vi "Test Save GIF (Memory).vi"(8 "error in (no error)":errorcluster) -> (0 "error out":errorcluster, 3 "Pass?":bool)   [LabVIEW 2020]
uses:
  <vilib>/picture/picture.llb/imagedata.ctl
  G-Image/Image IO/Polymorphic VIs/Save JPG Image (Memory).vi/70fca071-aecc-49e6-b287-23b8a0d46a54.vi
  G-Image/Private/Result To Error.vi
  G-Image/Private/Get Image Data.vi
  G-Image/Private/ARGB To RGBA.vi
  G-Image/Private/Depth To Number Channels.vi
  G-Image/Image Processing/Indexed Color To True Color Image.vi
  <vilib>/Utility/error.llb/Error Cluster From Error Code.vi
  G-Image/G-Image.lvlib
  G-Image/Image IO/Controls/Dither Type.ctl
  0a31d6d2-376c-4628-95d1-524ecda838ee.vi
  G-Image/Image IO/Polymorphic VIs/Save GIF Image (Path).vi
  G-Image/Image IO/Polymorphic VIs/Load Image (Path).vi
panel:
  out "Array":cluster{string, "new picture":picture}[](array[cluster])
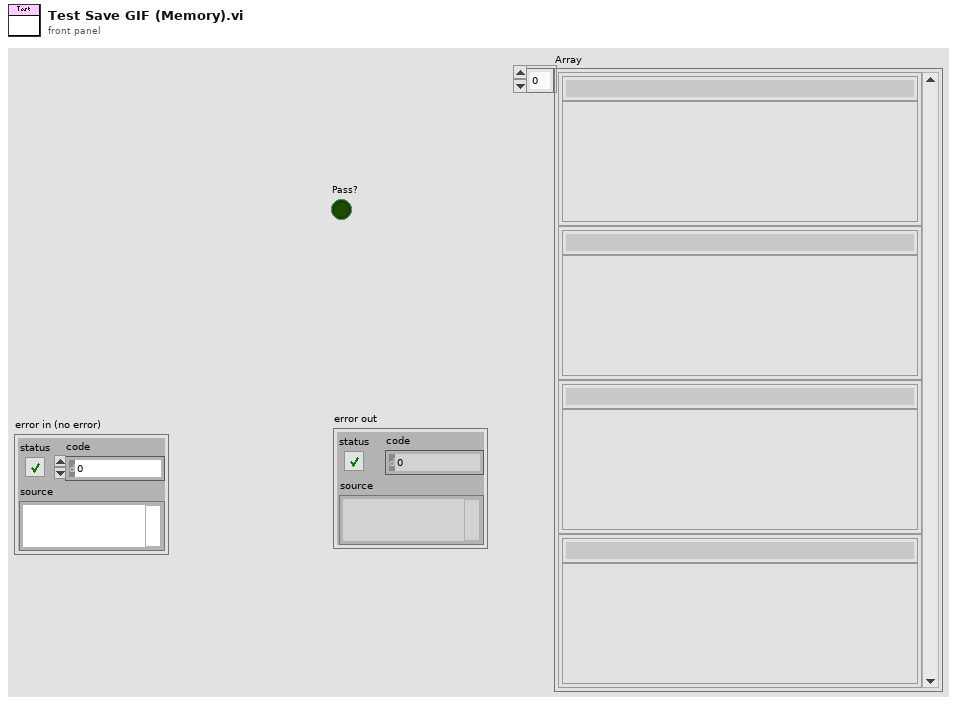
[diagram p1: front panel]
types:
  T1 = typedef "G-Image.lvlib/Dither Type.ctl" = enum32{"None", "Floyd-Steinberg"}
  T2 = typedef "imagedata.ctl" = cluster{"image type":i32, "image depth":i32, "image":u8[], "mask":u8[], "colors":u32[], "Rectangle":cluster{"left":i16, "top":i16, "right":i16, "bottom":i16}}
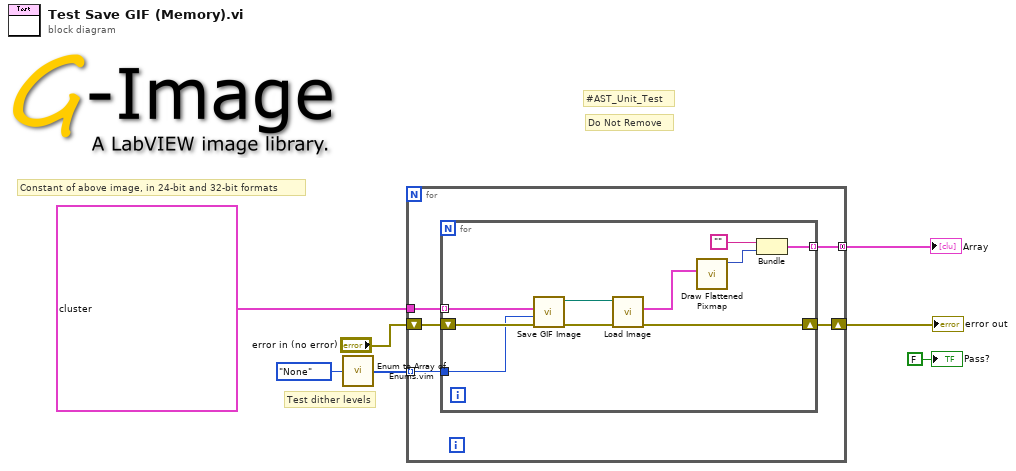
[diagram p0: block diagram]
diagram:
  # "Test dither levels"
  # "Constant of above image, in 24-bit and 32-bit formats"
  # "Do Not Remove"
  # "#AST_Unit_Test"
  n1 = call "Enum to Array of Enums.vim"("enum"=Dither_Type."None" ("Dither (None)")) -> ("array of enums"=w1:T1[])
  n2 = for {
    tunnel: [w11] -> w6 mode=concatenating
    tunnel: T2[] [{"image type"=0, "image depth"=24, "image"=array[115500 elements], "mask"=[], "colors"=[], "Rectangle"={"left"=0, "top"=0, "right"=350, "bottom"=110}}, {"image type"=0, "image depth"=32, "image"=array[154000 elements], "mask"=array[4840 elements], "colors"=[], "Rectangle"={"left"=0, "top"=0, "right"=350, "bottom"=110}}] ("Array 2") -> [w9]
    shift-right: [w10] -> w5
    shift-left: "error in (no error)" -> [w12]
    tunnel: w1 -> [w8] mode=indexing
    n3 = for {
      tunnel: w9 -> [w19] mode=indexing
      shift-right: [w14] -> w10
      shift-left: w12 -> [w22]
      tunnel: [w16] -> w11 mode=indexing
      tunnel: w8 -> [w13]
      n4 = call-poly "Save GIF Image.vi"("error in (no error)"=w22, "Dither (None)"=w13, "Image"=w19) -> ("error out"=w20:errorcluster, "Path Out"=w21:path)  [unwired: 7 in]
      n5 = call-poly "Load Image.vi"("error in (no error)"=w20, "Path In"=w21) -> ("error out"=w14:errorcluster, "Image"=w18:T2)  [unwired: 7 in, 1 out]
      n6 = call <vilib>:"Draw Flattened Pixmap.vi"("image data"=w18) -> ("new picture"=w17:picture)  [unwired: 8 in]
      n7 = Bundle("", "new picture"=w17) -> (w16:cluster{string, "new picture":picture})  [unwired: 1 in]
    }
  }
  "error out" <- w5
  "Array" <- w6
  "Pass?" <- FALSE ("Pass?")
